vi "SP click on control.vi"(7 "mySub":refnum<vi>, 8 "error in (no error)":errorcluster, 10 "Reference to Button":refnum<vi>, 11 "VI Reference":refnum<vi>) -> (0 "error out":errorcluster)   [LabVIEW 2020, in "ui-testing.lvlib"]
uses:
  ui-testing.lvlib
  User32.dll
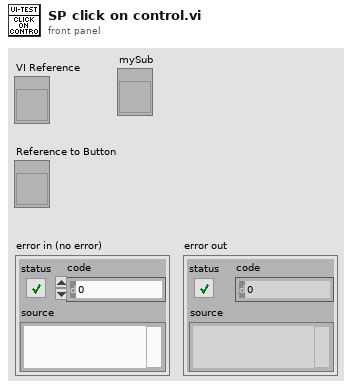
[diagram p1: front panel]
types:
  T1 = typedef "LVPositionTypeDef.ctl" = cluster{"Left":i32, "Top":i32}
  T2 = typedef "LVRectTypeDef.ctl" = cluster{"left":i16, "top":i16, "right":i16, "bottom":i16}
  T3 = typedef "LVPointTypeDef.ctl" = cluster{"Horizontal":i16, "Vertical":i16}
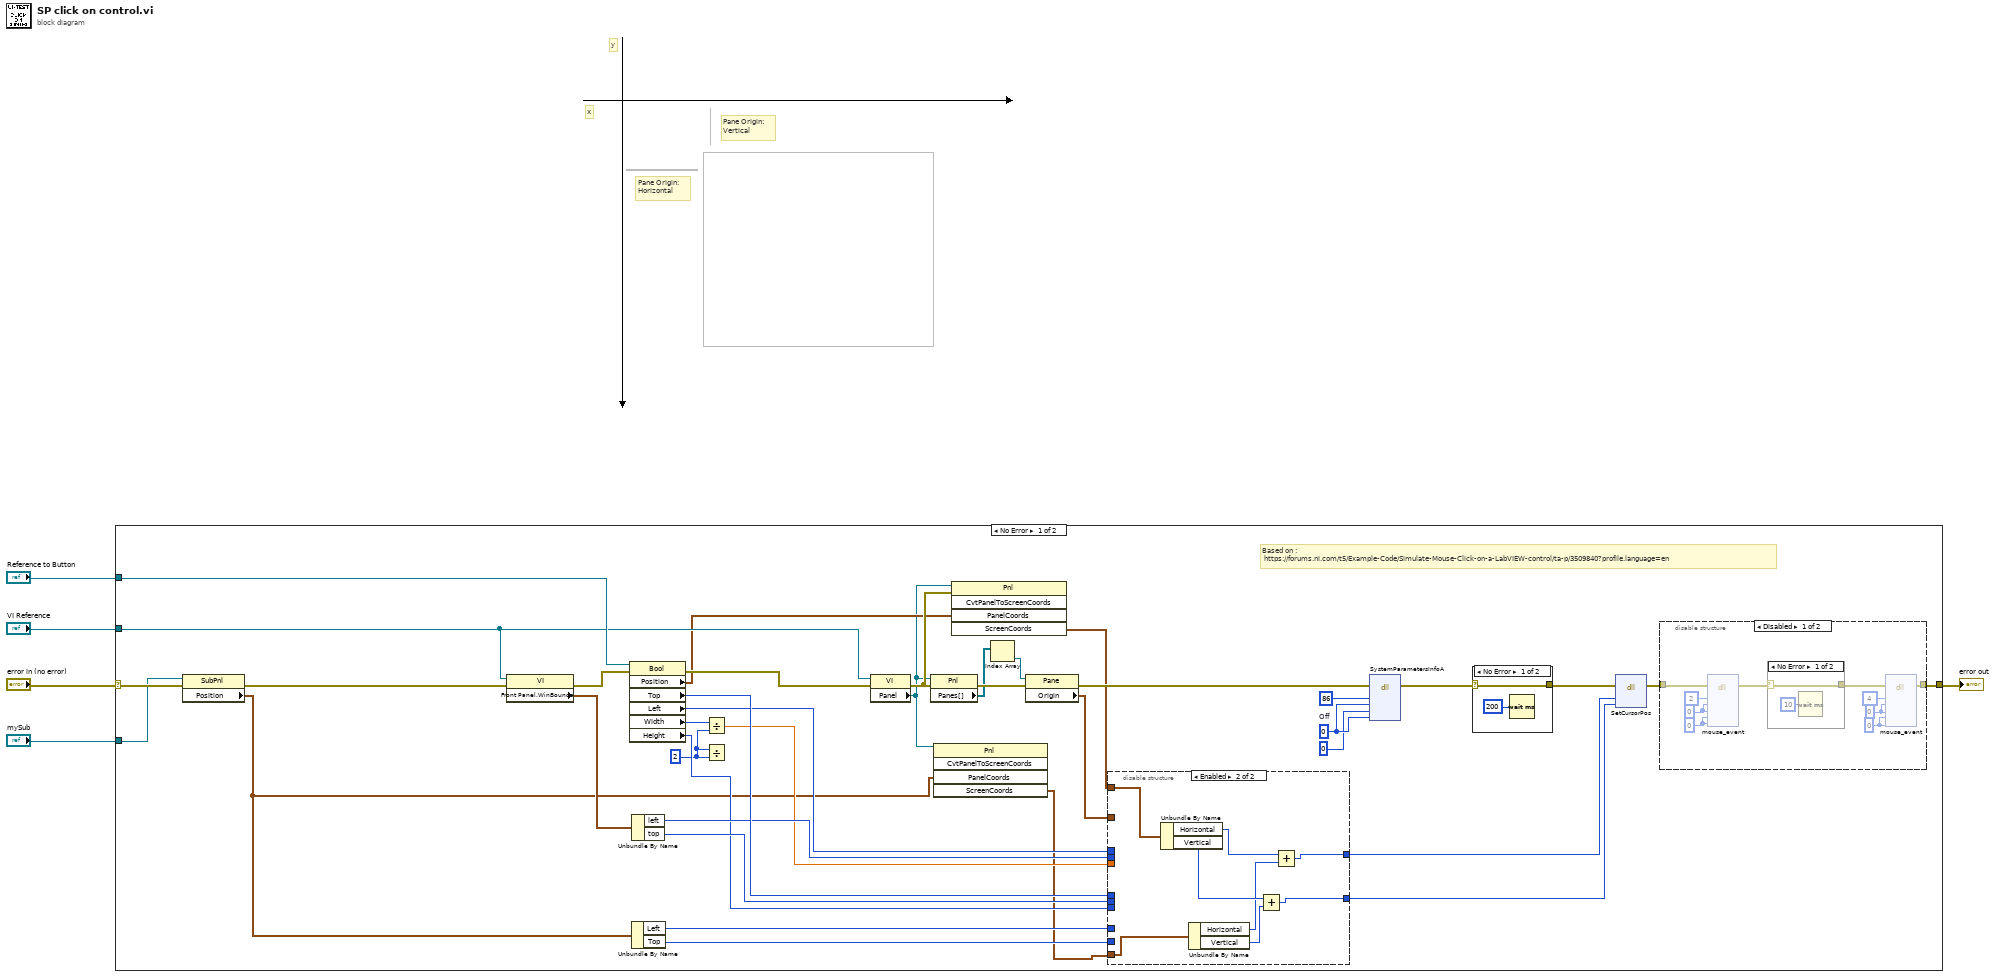
[diagram p0: block diagram]
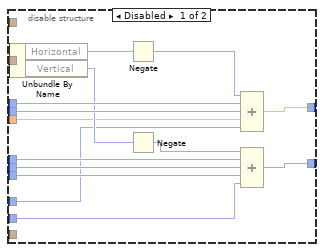
[diagram p4: hidden frame]
diagram:
  # "Pane Origin:\nVertical"
  # "Pane Origin:\nHorizontal"
  # "y"
  # "x"
  n1 = case shown="No Error" "error in (no error)" {
    selector: "error in (no error)" -> [w13 w83]
    tunnel: [w37 w83] -> w5
    tunnel: "Reference to Button" -> [w32 _]
    tunnel: "VI Reference" -> [w26 _]
    tunnel: "mySub" -> [w10 _]
    frame No Error {
      w17 = u32 2 ("y")
      w43 = u32 0  # Off
      # "Based on :\n https://forums.ni.com/t5/Example-Code/Simulate-Mouse-Click-on-a-LabVIEW-control/ta-p/3509840?profile.language=en"
      n2 = property class="SubPnl"(reference=w10, error in=w13) -> (error out=w9:errorcluster, "Position"=w7:T1)  [unwired: 1 out]
      n3 = property class="VI"(reference=w26, error in=w9) -> (error out=w28:errorcluster, "Front Panel.WinBounds"=w36:T2)  [unwired: 1 out]
      n4 = property on="Property Node" class="Bool"(reference=w32, error in=w28) -> (error out=w27:errorcluster, "Position"=w15:T1, "Top"=w35:i32, "Left"=w31:i32, "Width"=w20:u32, "Height"=w18:u32)  [unwired: 1 out]
      n5 = Unbundle By Name(w7) -> ("Left"=w12:i32, "Top"=w11:i32)
      n6 = Unbundle By Name(w36) -> ("left"=w30:i16, "top"=w34:i16)
      n7 = Divide(x=w20, y=w17) -> (x/y=w19:dbl)
      n8 = Divide(x=w17, y=w17) -> ()  [unwired: 1 out]
      n9 = property class="VI"(reference=w26, error in=w27) -> (error out=w16:errorcluster, "Panel"=w8:refnum<vi>)  [unwired: 1 out]
      n10 = property class="Pnl"(reference=w8, error in=w16) -> (error out=w25:errorcluster, "Panes[]"=w24:refnum<vi>[])  [unwired: 1 out]
      n11 = invoke class="Pnl" method="CvtPanelToScreenCoords"(reference=w8, "PanelCoords"=w7) -> ("ScreenCoords"=w6:T3)  [unwired: 3 in, 4 out]
      n12 = invoke class="Pnl" method="CvtPanelToScreenCoords"(reference=w8, error in=w16, "PanelCoords"=w15) -> ("ScreenCoords"=w14:T3)  [unwired: 2 in, 4 out]
      n13 = Index Array(array=w24) -> (element=w22:refnum<vi>)  [unwired: 1 in]
      n14 = property class="Pane"(reference=w22, error in=w25) -> (error out=w23:errorcluster, "Origin"=w21:T3)  [unwired: 1 out]
      n15 = disable-structure shown="Enabled" {
        disable-tunnel: w35 -> [w71 _]
        disable-tunnel: w34 -> [w70 _]
        disable-tunnel: [w69 w73] -> w33
        disable-tunnel: w31 -> [w68 _]
        disable-tunnel: w30 -> [w67 _]
        disable-tunnel: [w66 w75] -> w29
        disable-tunnel: w21 -> [w65 _]
        disable-tunnel: w19 -> [w60 _]
        disable-tunnel: w18 -> [w59 _]
        disable-tunnel: w14 -> [_ w79]
        disable-tunnel: w12 -> [w58 _]
        disable-tunnel: w11 -> [w57 _]
        disable-tunnel: w6 -> [_ w76]
        frame Disabled {
          n16 = Unbundle By Name(w65) -> ("Horizontal"=w64:i16, "Vertical"=w63:i16)
          n17 = Negate(x=w64) -> (-x=w62:i16)
          n18 = Negate(x=w63) -> (-x=w61:i16)
          n19 = Compound Arithmetic op=ADD(w62, w68, w67, w60, w58) -> (w66:dbl)
          n20 = Compound Arithmetic op=ADD(w61, w71, w70, w59, w57) -> (w69:u32)
        }
        frame Enabled {
          n21 = Unbundle By Name(w79) -> ("Horizontal"=w78:i16, "Vertical"=w77:i16)
          n22 = Unbundle By Name(w76) -> ("Horizontal"=w74:i16, "Vertical"=w72:i16)
          n23 = Add(x=w77, y=w72) -> (x+y=w73:i16)
          n24 = Add(x=w78, y=w74) -> (x+y=w75:i16)
        }
      }
      n25 = dll-call lib="User32.dll" fn="SystemParametersInfoA" label="Terminate power-off mode"(error in=w23, "uiAction"=u32 86 ("SPI_GETPOWEROFFACTIVE"), "uiParam"=w43, "pvParam"=0, "fWinIni"=w43) -> (error out=w40:errorcluster)  [unwired: 7 in, 1 out]
      n26 = case shown="No Error" w40 {
        selector: w40 -> [w80 w82]
        tunnel: [w80 w82] -> w39
        frame No Error {
          n27 = Wait (ms)(milliseconds to wait=u32 200) -> ()  [unwired: 1 out]
        }
        frame Error {
        }
      }
      n28 = dll-call lib="User32.dll" fn="SetCursorPos" label="Move mouse"(error in=w39, "dx"=w29, "dy"=w33) -> (error out=w38:errorcluster)  [unwired: 5 in, 1 out]
      n29 = disable-structure shown="Disabled" {
        disable-tunnel: w38 -> [w47 _]
        disable-tunnel: [w44 _] -> w37
        frame Disabled {
          w51 = 0 ("dwExtraInfo")
          w52 = u32 0 ("dwExtraInfo")
          w50 = 0 ("dwExtraInfo")
          w49 = u32 0 ("dwExtraInfo")
          n30 = dll-call lib="User32.dll" fn="mouse_event" label="Click"(error in=w47, "dwFlags"=2, "dx"=w50, "dy"=w50, "dwData"=w49, "dwExtraInfo"=w49) -> (error out=w46:errorcluster)  [unwired: 8 in, 1 out]
          n31 = case shown="No Error" w46 {
            selector: w46 -> [w54 w56]
            tunnel: [w54 w56] -> w45
            frame No Error {
              n32 = Wait (ms)(milliseconds to wait=u32 10) -> ()  [unwired: 1 out]
            }
            frame Error {
            }
          }
          n33 = dll-call lib="User32.dll" fn="mouse_event" label="Release"(error in=w45, "dwFlags"=4, "dx"=w51, "dy"=w51, "dwData"=w52, "dwExtraInfo"=w52) -> (error out=w44:errorcluster)  [unwired: 8 in, 1 out]
        }
        frame Enabled {
        }
      }
    }
    frame Error {
    }
  }
  "error out" <- w5
